vi "AIbool_tt.vi"() -> (0 "AIarray":bool[](array[boolean]), 2 "Sigcase":i16)   [LabVIEW 2013]
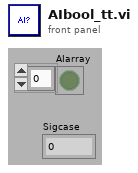
[diagram p1: front panel]
types:
  T1 = cluster{"StageS":i32, "StageL":i32, "data dir":path, "image OD":u16, "contour OD":u16, "point OD":u16, "AOlines":tag[], "AIlines":tag[], "CI lines":tag[], "DO lines":tag[], "AO names":string[], "CI names":string[], "AI names":string[], "DO names":string[], "CIextensions":string[], "AIextensions":string[], "Voltage to Ygalvo":i32, "Voltage to Xgalvo":i32, "Voltage to patch":i32, "640 shutter":i32, "2P shutter":i32, "LT timestamp":i32, "Vp":i32, "Ip":i32}
  T2 = typedef "LVRectTypeDef.ctl" = cluster{"Left":i16, "Top":i16, "Right":i16, "Bottom":i16}
  T3 = cluster{"Xpixels":i32, "Vxminref":dbl, "Vxmaxref":dbl, "P":dbl, "Ypixels":i32, "Vyminref":dbl, "Vymaxref":dbl, "srate":sgl, "sAOxy":i32, "timeout":dbl, "type":string, "date":string, "time":string, "Colormap":u16, "Drawing Mode":u16, "Scanning Mode":u16, "square pixels":bool, "square matrix":bool, "Xpixels Img":i32, "Vx-min Img":dbl, "VX-max Img":dbl, "Ypixels Img":i32, "Vy-min Img":dbl, "Vy-max Img ":dbl, "Angle Img":dbl, "autoshutter":bool, "finite":bool, "cont":bool, "wavdet":bool, "measpoints":i32, "avpp":i32, "bufferAO":i32, "bufferAI":i32, "starttick":u32, "waveform":path, "Vx-ref":dbl, "Vy-ref":dbl, "refreshrate":dbl, "refreshbuffer":i32, "tt_cycles":i32, "motorref":refnum<k7>, "mirrorswitch":refnum<k7>, "sample mode":i32, "maxbufferAI":i32, "sampletreshold":dbl, "srateAODO":sgl, "bin":sgl, "Pel":sgl, "Angle draw":dbl, "srate Img":sgl, "ROIimg_plotbounds":T2, "auto OD":bool, "ODfilt":u16, "reset AO_DO":bool, "aAI":i32[], "aCI":i32[], "aAO":i32[], "aDO":i32[]}
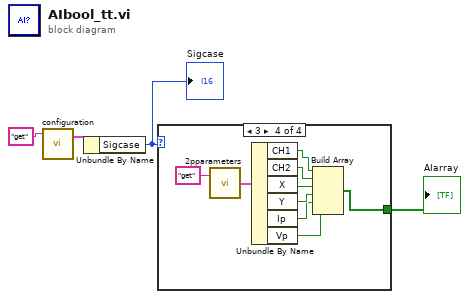
[diagram p0: block diagram]
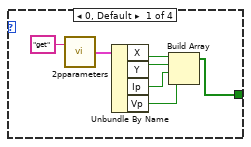
[diagram p2: hidden frame]
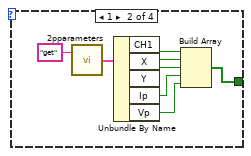
[diagram p3: hidden frame]
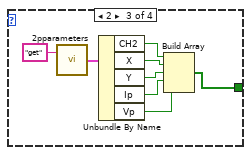
[diagram p4: hidden frame]
diagram:
  n1 = call "configuration.vi"("command"="get") -> ("config out"=w4:T1)  [unwired: 2 in, 1 out]
  n2 = Unbundle By Name(w4) -> ("Sigcase"=w1:i16)
  "Sigcase" <- w1
  n3 = case shown="3" w1 {
    tunnel: [w7 w14 w22 w30] -> w2
    frame 0, Default {
      n4 = call "2pparameters.vi"("command"="get") -> ("params out"=w11:T3)  [unwired: 1 in]
      n5 = Unbundle By Name(w11) -> ("X"=w9:bool, "Y"=w8:bool, "Ip"=w6:bool, "Vp"=w5:bool)
      n6 = Build Array(w9, w8, w6, w5) -> (w7:bool[])
    }
    frame 1 {
      n7 = call "2pparameters.vi"("command"="get") -> ("params out"=w19:T3)  [unwired: 1 in]
      n8 = Unbundle By Name(w19) -> ("CH1"=w17:bool, "X"=w16:bool, "Y"=w15:bool, "Ip"=w13:bool, "Vp"=w12:bool)
      n9 = Build Array(w17, w16, w15, w13, w12) -> (w14:bool[])
    }
    frame 2 {
      n10 = call "2pparameters.vi"("command"="get") -> ("params out"=w27:T3)  [unwired: 1 in]
      n11 = Unbundle By Name(w27) -> ("CH2"=w25:bool, "X"=w24:bool, "Y"=w23:bool, "Ip"=w21:bool, "Vp"=w20:bool)
      n12 = Build Array(w25, w24, w23, w21, w20) -> (w22:bool[])
    }
    frame 3 {
      n13 = call "2pparameters.vi"("command"="get") -> ("params out"=w36:T3)  [unwired: 1 in]
      n14 = Unbundle By Name(w36) -> ("CH1"=w34:bool, "CH2"=w33:bool, "X"=w32:bool, "Y"=w31:bool, "Ip"=w29:bool, "Vp"=w28:bool)
      n15 = Build Array(w34, w33, w32, w31, w29, w28) -> (w30:bool[])
    }
  }
  "AIarray" <- w2
